vi "DraggingDresser.vi"() -> ()   [LabVIEW 2014]
doc: "This program takes a coefficient of friction input and models the problem of pulling a dresser at an angle.\nThe program outputs a graph of the force per unit weight from 0 to 90 degrees. The force for a given angle\ncan also be retrieved and the angle of minimum force required to move the dresser is also reported.\n\nBryan Ghahremani - SID: 1135515\nKenneth Heide - SID: 1269429"
panel:
  out "Force":dbl[](array[numeric])
  out "Angle for Minimum Force":i32 format="%.1f"
  in  "Coefficient of Kinetic Friction":dbl format="%.1f"
  out "Waveform Graph":dbl[](graph)
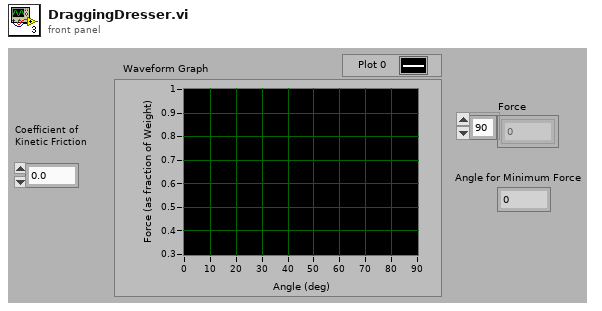
[diagram p1: front panel]
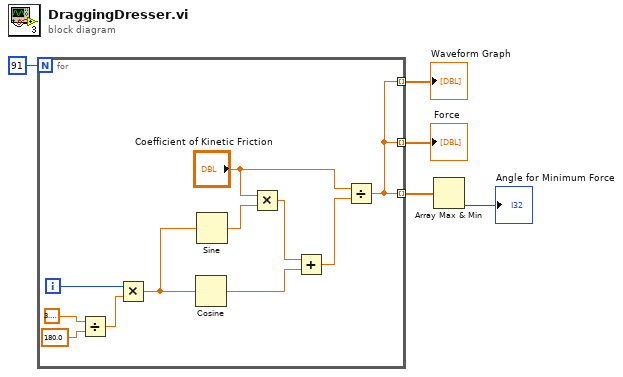
[diagram p0: block diagram]
diagram:
  n1 = for {
    N: 91 -> [_]
    tunnel: [w6] -> w4 mode=indexing
    tunnel: [w6] -> w1 mode=indexing
    tunnel: [w6] -> w2 mode=indexing
    i -> [w16]
    n2 = Divide(x=3.141592653589793, y=180.0) -> (x/y=w13:dbl)
    n3 = Multiply(x=w16, y=w13) -> (x*y=w12:dbl)
    n4 = Cosine(x=w12) -> (cos(x)=w9:dbl)
    n5 = Sine(x=w12) -> (sin(x)=w11:dbl)
    n6 = Multiply(x="Coefficient of Kinetic Friction", y=w11) -> (x*y=w10:dbl)
    n7 = Add(x=w10, y=w9) -> (x+y=w7:dbl)
    n8 = Divide(x="Coefficient of Kinetic Friction", y=w7) -> (x/y=w6:dbl)
  }
  "Waveform Graph" <- w2
  "Force" <- w1
  n9 = Array Max & Min(array=w4) -> (min index (indices)=→"Angle for Minimum Force":i32)  [unwired: 3 out]
